vi "测试-腐蚀图片.vi"() -> ()   [LabVIEW 2018]
uses:
  <vilib>/vision/NI_Vision_Development_Module.lvlib
panel:
  in  "Structuring Element":i32[][](array[numeric])=[[1, 1, 1], [1, 1, 1], [1, 1, 1]]
  out "处理后 2":T1(plugin-control)
  in  "Operation":T2(ring)
  in  "腐蚀大小":i32=3
  out "原图":T1(plugin-control)
  out "处理后":T1(plugin-control)
  out "标注图":T1(plugin-control)
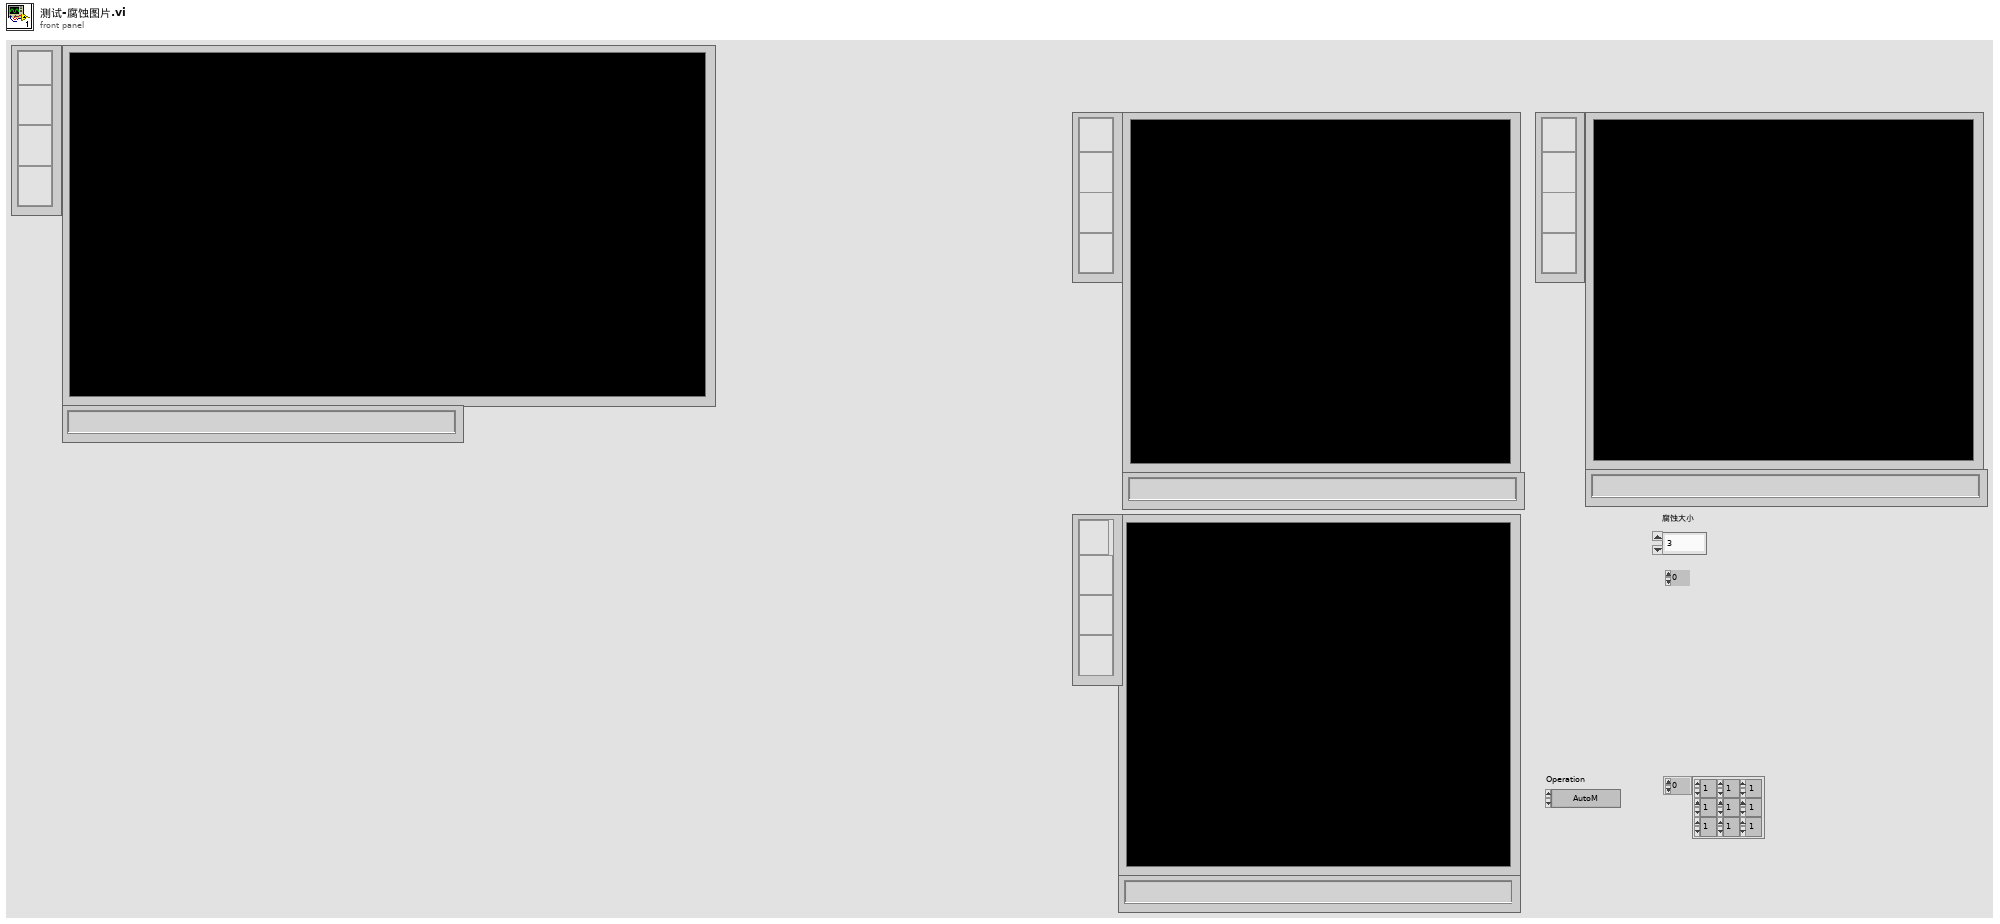
[diagram p1: front panel]
types:
  T1 = typedef "IMAQ Image.ctl" = refnum<image>
  T2 = enum32{"AutoM", "Close", "Dilate", "Erode", "Gradient", "Gradient in", "Gradient out", "HitMiss", "Open", "PClose", "POpen", "Thick", "Thin"}
  T3 = typedef "Image Type" = u32
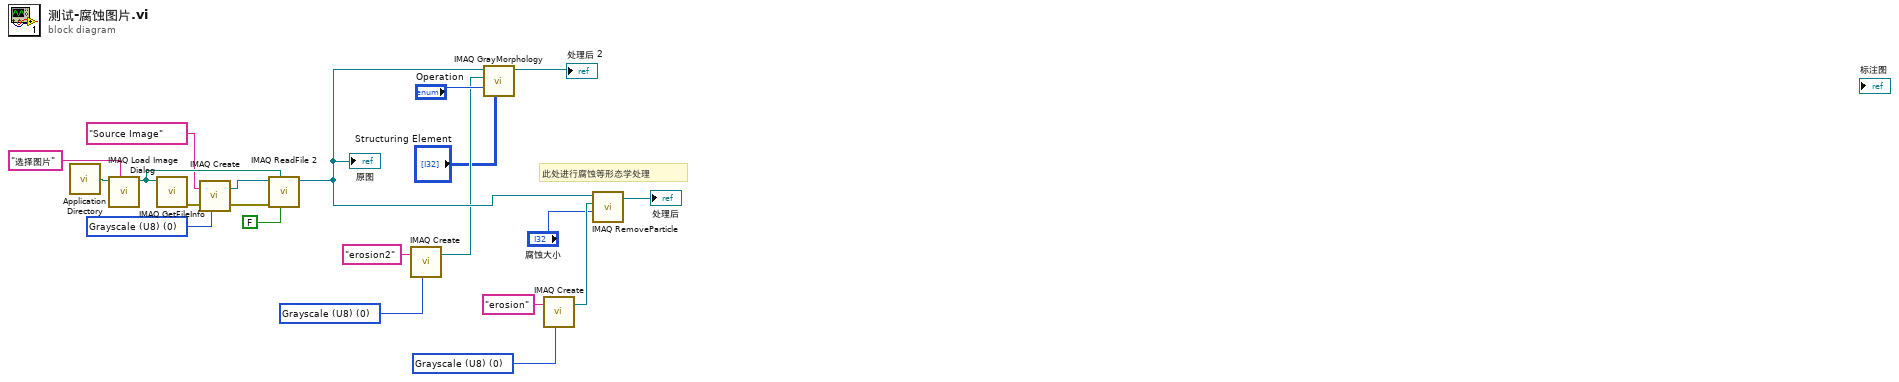
[diagram p0: block diagram]
diagram:
  w4 = T3 0 items=["Grayscale (U8)", "Grayscale (I16)", "Grayscale (SGL)", "Complex (CSG)", "RGB (U32)", "HSL (U32)", "RGB (U64)", "Grayscale (U16)"] ("Image Type")
  w10 = T3 0 items=["Grayscale (U8)", "Grayscale (I16)", "Grayscale (SGL)", "Complex (CSG)", "RGB (U32)", "HSL (U32)", "RGB (U64)", "Grayscale (U16)"] ("Image Type")
  w21 = T3 0 items=["Grayscale (U8)", "Grayscale (I16)", "Grayscale (SGL)", "Complex (CSG)", "RGB (U32)", "HSL (U32)", "RGB (U64)", "Grayscale (U16)"] ("Image Type")
  # "此处进行腐蚀等形态学处理"
  n1 = call <vilib>:"Application Directory.vi"() -> ("Application Directory"=w18:path)
  n2 = call "IMAQ Load Image Dialog"("Prompt"="选择图片" ("prompt"), "Start Path"=w18) -> ("Path"=w14:path)  [unwired: 7 in, 2 out]
  n3 = call "IMAQ GetFileInfo"("File Path"=w14) -> ("error out"=w15:errorcluster)  [unwired: 4 in, 6 out]
  n4 = call "IMAQ Create"("Image Name"="Source Image", "Image Type"=w10, "error in (no error)"=w15) -> ("New Image"=w16:T1, "error out"=w17:errorcluster)  [unwired: 2 in]
  n5 = call "IMAQ ReadFile 2"("Use File Path Image Type"=FALSE, "File Path"=w14, "error in (no error)"=w17, "Image"=w16) -> ("Image Out"=w7:T1)  [unwired: 3 in, 4 out]
  "原图" <- w7
  n6 = call "IMAQ Create"("Image Name"="erosion2", "Image Type"=w4) -> ("New Image"=w2:T1)  [unwired: 3 in, 1 out]
  n7 = call "IMAQ GrayMorphology"("Structuring Element"="Structuring Element", "Operation"="Operation", "Image Dst"=w2, "Image Src"=w7) -> ("Image Dst Out"=→"处理后 2":T1)  [unwired: 6 in, 1 out]
  n8 = call "IMAQ Create"("Image Name"="erosion", "Image Type"=w21) -> ("New Image"=w19:T1)  [unwired: 3 in, 1 out]
  n9 = call "IMAQ RemoveParticle"("Number of Erosion"="腐蚀大小", "Image Dst"=w19, "Image Src"=w7) -> ("Image Dst Out"=→"处理后":T1)  [unwired: 7 in, 1 out]
